vi "UserInterface.vi"(10 "Published Data":string[][](array[string]), 11 "Display Cluster Input":refnum<vi>) -> ()   [LabVIEW 2015]
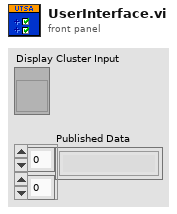
[diagram p1: front panel]
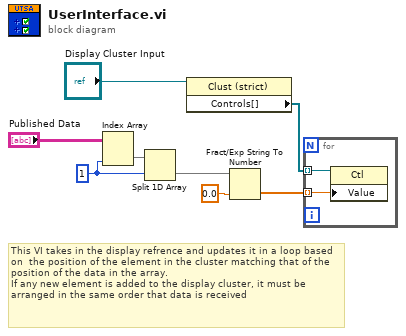
[diagram p0: block diagram]
diagram:
  w7 = 1 ("disabled index (col)")
  # "This VI takes in the display refrence and updates it in a loop based on  the position of the element in the cluster matching that of the position of the data in the array.  \nIf any new element is added to the display cluster, it must be arranged in the same order that data is received"
  n1 = Index Array(array="Published Data", index (col)=w7) -> (element=w6:string[])  [unwired: 1 in]
  n2 = Split 1D Array(array=w6, index=w7) -> (second subarray=w8:string[])  [unwired: 1 out]
  n3 = property class="Clust (strict)"(reference="Display Cluster Input") -> ("Controls[]"=w1:refnum<vi>[])  [unwired: 1 in, 2 out]
  n4 = Fract/Exp String To Number(string=w8, default (0 dbl)=0.0 ("default (0 DBL)")) -> (number=w2:dbl[])  [unwired: 2 in, 1 out]
  n5 = for {
    tunnel: w2 -> [w9] mode=indexing
    tunnel: w1 -> [w10] mode=indexing
    n6 = property class="Ctl"(reference=w10, "Value"=w9) -> ()  [unwired: 1 in, 2 out]
  }
